vi "View license.vi"() -> ()   [LabVIEW 2009]
panel:
  out "String":string
  in  "stop":bool
  # "Copyright 2009, 2010, 2011 Martin Persson \n   martin.persson@physics.gu.se"
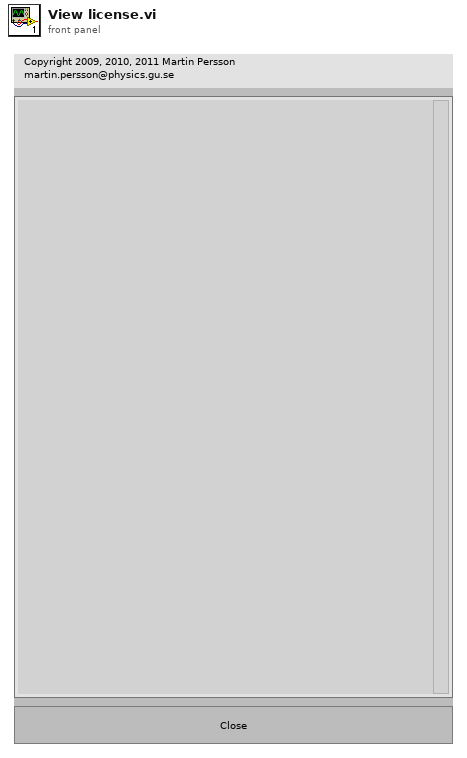
[diagram p1: front panel]
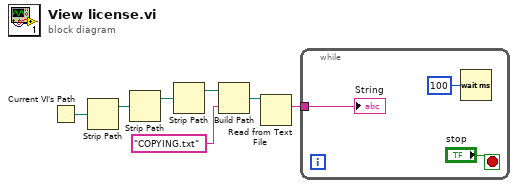
[diagram p0: block diagram]
diagram:
  n1 = Current VI's Path() -> (path=w6:path)
  n2 = Strip Path(path=w6) -> (stripped path=w5:path)  [unwired: 1 out]
  n3 = Strip Path(path=w5) -> (stripped path=w3:path)  [unwired: 1 out]
  n4 = Strip Path(path=w3) -> (stripped path=w2:path)  [unwired: 1 out]
  n5 = Build Path(base path=w2, name or relative path="COPYING.txt") -> (appended path=w4:path)
  n6 = Read from Text File(file (use dialog)=w4) -> (text=w1:string)  [unwired: 3 in, 3 out]
  n7 = while {
    tunnel: w1 -> [w10]
    stop <- "stop" stop-if-true
    n8 = Wait (ms)(milliseconds to wait=u32 100) -> ()  [unwired: 1 out]
    "String" <- w10
  }
